vi "CDhb.vi"(1 "Vehicle Volume (Vm)":dbl, 2 "dcp/dx":dbl, 3 "Vehicle Frontal Area (Am)":dbl) -> (0 "Numeric":dbl)   [LabVIEW 2017]
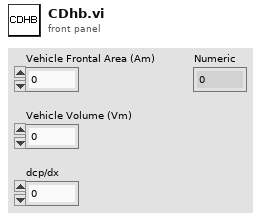
[diagram p1: front panel]
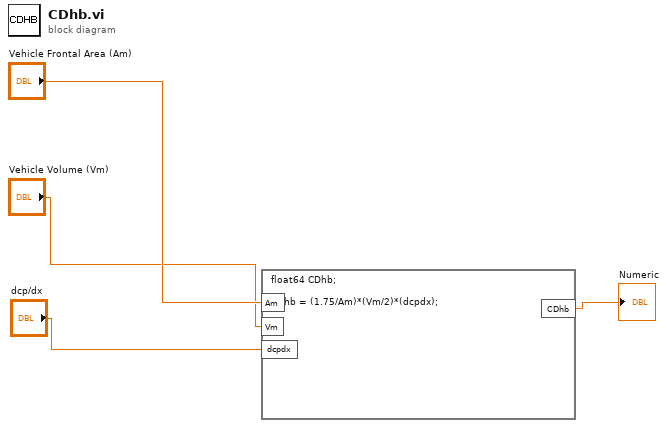
[diagram p0: block diagram]
diagram:
  n1 = formula code="float64 CDhb;\n\nCDhb = (1.75/Am)*(Vm/2)*(dcpdx);"("Am"="Vehicle Frontal Area (Am)", "Vm"="Vehicle Volume (Vm)", "dcpdx"="dcp/dx") -> ("CDhb"=→"Numeric":dbl)
